vi "DAQmxTaskContainerMoveCrystal-Com-Exec.vi"(8 "error in (no error)":errorcluster, 9 "data":variant, 10 "ControlQueue":refnum<queue>, 11 "DAQmxTaskContainer in":refnum<class "DAQmxTaskContainer.lvclass">) -> (0 "error out":errorcluster, 3 "DAQmxTaskContainer out":refnum<class "DAQmxTaskContainer.lvclass">)   [LabVIEW 2015, in "DAQmxTaskContainer.lvclass"]
uses:
  DAQmxTaskContainer.lvclass
  dependecies/ControlsVIs/Clusters-def/SERVER-Commands.ctl
  dependecies/ControlsVIs/Clusters-def/ProtypeCommand-DAQmxReply.ctl
  DAQmxTask.lvclass
  Control/Control-Server/Control-Server.lvclass
  DAQmxTaskContainer_General/DAQmxTaksContainer_General.lvclass
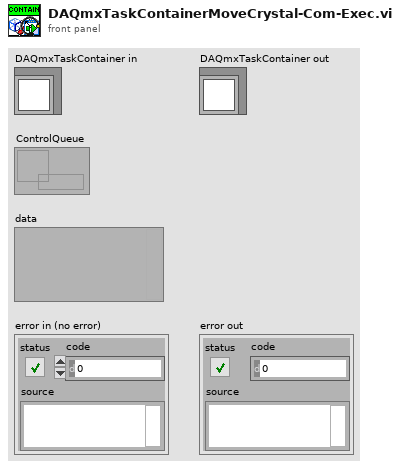
[diagram p1: front panel]
types:
  T1 = typedef "ProtypeCommand-DAQmxReply.ctl" = cluster{"On/Off":bool, "error out":errorcluster}
  T2 = typedef "Control-Server.lvclass/SERVER-Commands.ctl" = string
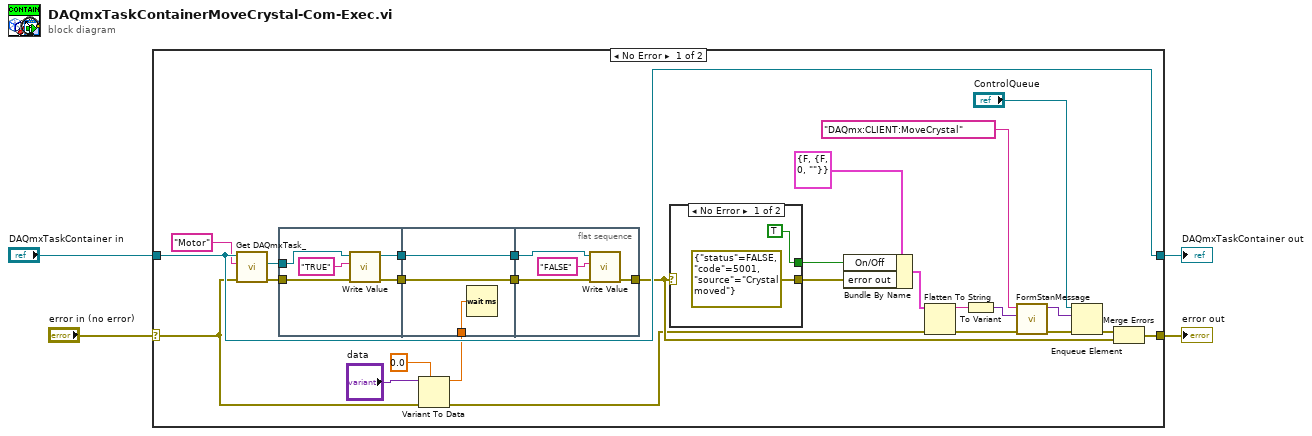
[diagram p0: block diagram]
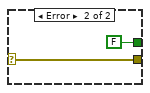
[diagram p2: hidden frame]
diagram:
  n1 = case shown="No Error" "error in (no error)" {
    selector: "error in (no error)" -> [w27 w49]
    tunnel: [w30 w48] -> w4
    tunnel: [w29 w49] -> w3
    tunnel: "DAQmxTaskContainer in" -> [w30 w48]
    frame No Error {
      n2 = call "Get DAQmxTask_.vi"("error in (no error)"=w27, "Task name"="Motor", "DAQmxTaksContainer_General in"=w30) -> ("error out"=w21:errorcluster, "DAQmx Task"=w19:refnum<class "DAQmxTask.lvclass">)  [unwired: 6 in, 1 out]
      n3 = flat-sequence {
        tunnel: w21 -> [w40]
        tunnel: w19 -> [w38]
        tunnel: [w37] -> w26
        tunnel: [w36] -> w25
        tunnel: [w43] -> w24
        tunnel: w26 -> [w43]
        tunnel: w18 -> [w42]
        tunnel: [w41] -> w23
        tunnel: w25 -> [w41]
        tunnel: w24 -> [w47]
        tunnel: w23 -> [w46]
        tunnel: [w45] -> w17
        frame #0 {
          n4 = call-dynamic "Write Value.vi"("error in (no error)"=w40, "Data"="TRUE", "DAQmxTask en entrée"=w38) -> ("error out"=w36:errorcluster, "DAQmxTask en sortie"=w37:refnum<class "DAQmxTask.lvclass">)  [unwired: 7 in]
        }
        frame #1 {
          n5 = Wait (ms)(milliseconds to wait=w42) -> ()  [unwired: 1 out]
        }
        frame #2 {
          n6 = call-dynamic "Write Value.vi"("error in (no error)"=w46, "Data"="FALSE", "DAQmxTask en entrée"=w47) -> ("error out"=w45:errorcluster)  [unwired: 7 in, 1 out]
        }
      }
      n7 = Variant To Data(error in=w27, type=0.0, Variant="data") -> (data=w18:dbl, error out=w11:errorcluster)
      n8 = case shown="No Error" w17 {
        selector: w17 -> [_ w35]
        tunnel: [errorcluster {"status"=FALSE, "code"=5001, "source"="Crystal moved"} ("error constant") w35] -> w15
        tunnel: [TRUE FALSE] -> w14
        frame No Error {
        }
        frame Error {
        }
      }
      n9 = Bundle By Name(cluster=T1 {"On/Off"=FALSE, "error out"={"status"=FALSE, "code"=0, "source"=""}} ("output cluster"), "On/Off"=w14, "error out"=w15) -> (w13:T1)
      n10 = Flatten To String(anything=w13, error in (no error)=w11) -> (data string=w12:string, error out=w6:errorcluster)  [unwired: 2 in, 1 out]
      n11 = To Variant(anything=w12) -> (Variant=w8:variant)
      n12 = call "FormStanMessage.vi"("error in"=w6, "data"=w8, "Command"=T2 "DAQmx:CLIENT:MoveCrystal" ("command")) -> ("error out"=w5:errorcluster, "message"=w7:variant)  [unwired: 7 in]
      n13 = Enqueue Element(queue="ControlQueue", element=w7, error in (no error)=w5) -> (error out=w10:errorcluster)  [unwired: 1 in, 2 out]
      n14 = Merge Errors(w10, w17) -> (w29:errorcluster)
    }
    frame Error {
    }
  }
  "DAQmxTaskContainer out" <- w4
  "error out" <- w3
